vi "Object_Create.vi"(8 "error in (no error)":errorcluster, 10 "Object Attributes":T1, 11 "Object In":refnum<class "Object.lvclass">) -> (0 "error out":errorcluster, 3 "Object Out":refnum<class "Object.lvclass">)   [LabVIEW 2017, in "Front Panel Publisher.lvlib" / "Object.lvclass"]
uses:
  Object.lvclass
  Web Front Panel_class/Web Front Panel.lvclass
  Coordinates.ctl
  Attributes.ctl
  <vilib>/Utility/miscctls.llb/LVRectTypeDef.ctl
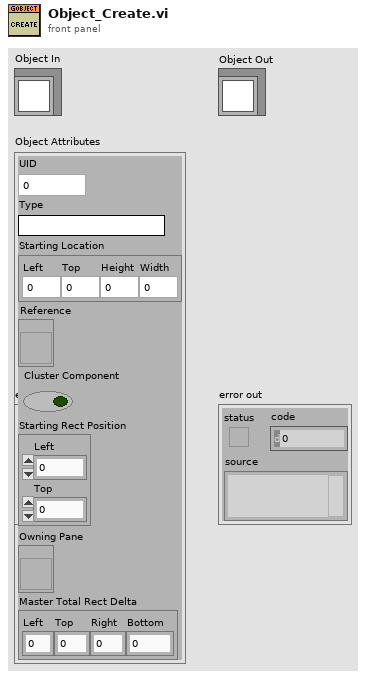
[diagram p1: front panel]
types:
  T1 = typedef "Front Panel Publisher.lvlib/Object.lvclass/Attributes.ctl" = cluster{"UID":i32, "Type":string, "Starting Location":T2, "Reference":refnum<vi>, "Cluster Component":bool, "Starting Rect Position":cluster{"Left":i16, "Top":i16}, "Owning Pane":refnum<vi>, "Master Total Rect Delta":T3}
  T2 = typedef "Front Panel Publisher.lvlib/Object.lvclass/Coordinates.ctl" = cluster{"Left":i32, "Top":i32, "Height":u32, "Width":u32}
  T3 = typedef "LVRectTypeDef.ctl" = cluster{"Left":i16, "Top":i16, "Right":i16, "Bottom":i16}
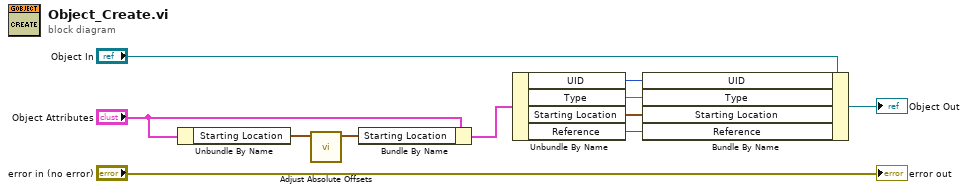
[diagram p0: block diagram]
diagram:
  n1 = Unbundle By Name("Object Attributes") -> ("Starting Location"=w7:T2)
  n2 = call "Adjust Absolute Offsets.vi"("Coordinates in"=w7) -> ("Coordinates out"=w6:T2)  [unwired: 8 in, 2 out]
  n3 = Bundle By Name(cluster="Object Attributes", "Starting Location"=w6) -> (w5:T1)
  n4 = Unbundle By Name(w5) -> ("UID"=w4:i32, "Type"=w3:string, "Starting Location"=w2:T2, "Reference"=w1:refnum<vi>)
  n5 = Bundle By Name(cluster="Object In", "UID"=w4, "Type"=w3, "Starting Location"=w2, "Reference"=w1) -> (→"Object Out":refnum<class "Object.lvclass">)
  "error out" <- "error in (no error)"
